vi "Communication_Handler.vi"() -> ()   [LabVIEW 2016]
panel:
  out "name (unnamed)":string
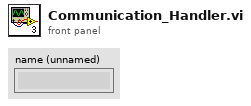
[diagram p1: front panel]
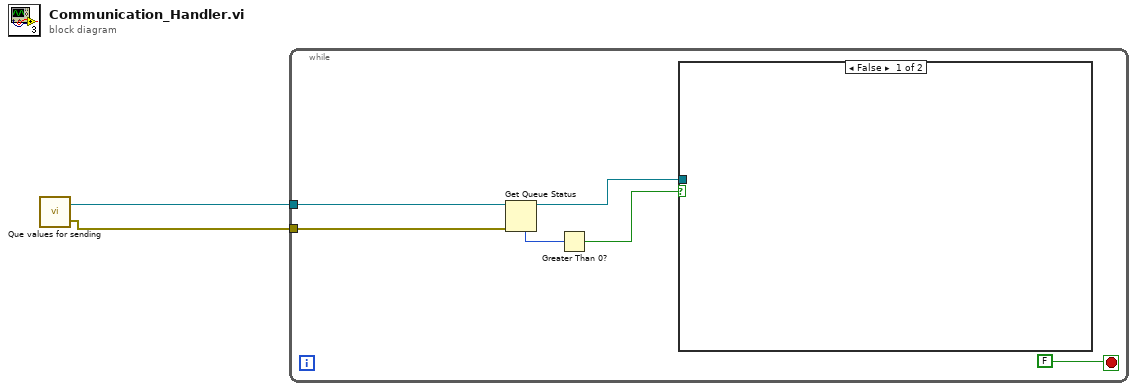
[diagram p0: block diagram]
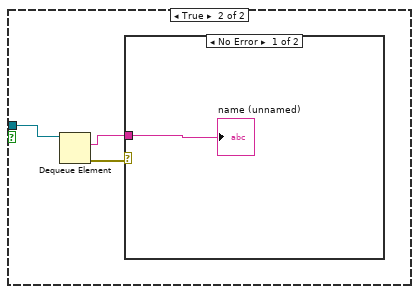
[diagram p2: hidden frame]
diagram:
  n1 = call "Que values for sending.vi"() -> ("error out"=w1:errorcluster, "queue out"=w2:refnum<queue>)  [unwired: 2 in]
  n2 = while {
    tunnel: w2 -> [w4]
    tunnel: w1 -> [w3]
    stop <- FALSE stop-if-true
    n3 = Get Queue Status(queue=w4, error in (no error)=w3) -> (queue out=w8:refnum<queue>, # elements in queue=w7:i32)  [unwired: 1 in, 6 out]
    n4 = Greater Than 0?(x=w7) -> (x > 0?=w6:bool)
    n5 = case shown="False" w6 {
      tunnel: w8 -> [_ w9]
      frame False {
      }
      frame True {
        n6 = Dequeue Element(queue=w9) -> (element=w10:string, error out=w11:errorcluster)  [unwired: 2 in, 2 out]
        n7 = case shown="No Error" w11 {
          tunnel: w10 -> [w12 _]
          frame No Error {
            "name (unnamed)" <- w12
          }
          frame Error {
          }
        }
      }
    }
  }
